vi "Lefoo Atmospheric pressure.vi"(8 "错误输入（无错误）":errorcluster, 11 "VISA resource name":refnum<visa-resource-name> caption="VISA") -> (0 "error out":errorcluster caption="错误输出", 1 "data":string, 2 "Atmospheric pressure":dbl)   [LabVIEW 2017]
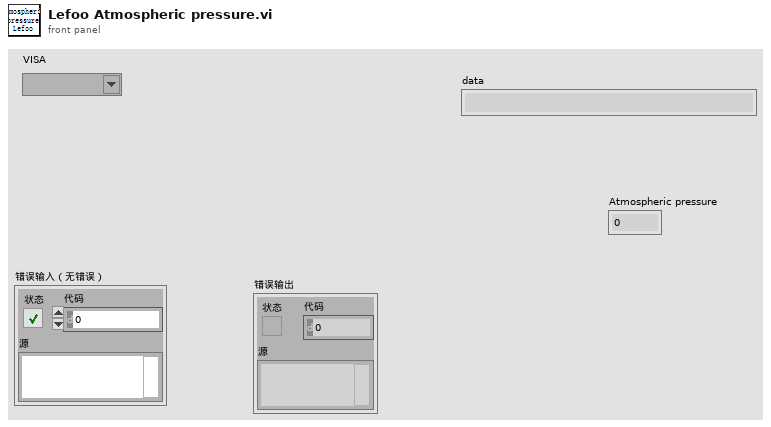
[diagram p1: front panel]
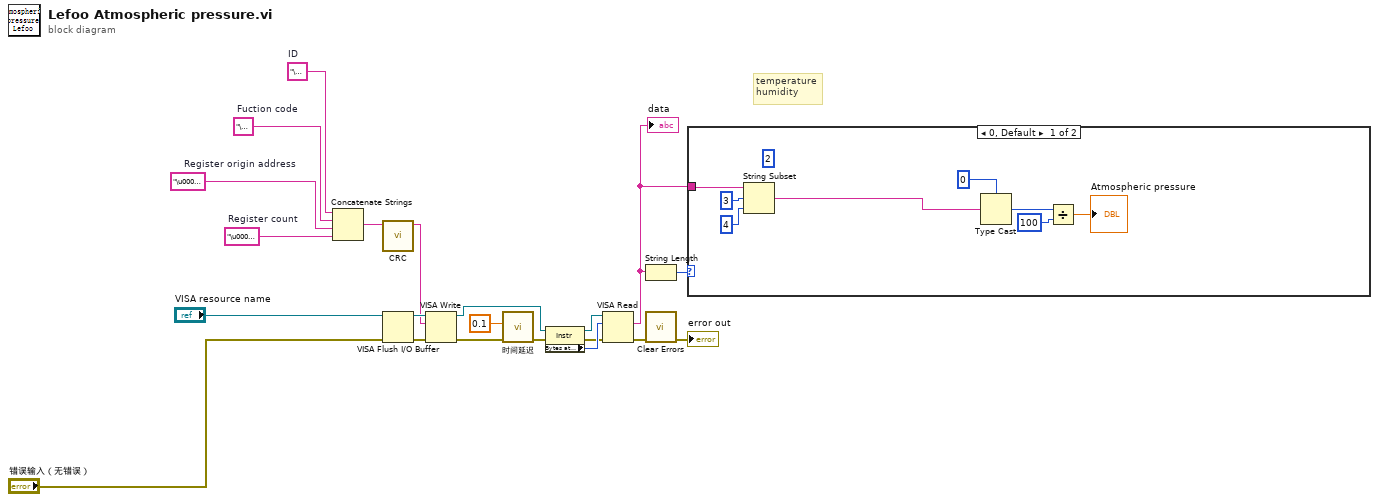
[diagram p0: block diagram]
diagram:
  w2 = "\u0000\u0001"  # Register count
  w4 = "\u0000\u0000"  # Register origin address
  w5 = "\u0003"  # Fuction code
  w6 = "\u0001"  # ID
  # "temperature\nhumidity"
  n1 = Concatenate Strings(w6, w5, w4, w2) -> (w3:string)
  n2 = call "CRC.vi"("字符串"=w3) -> ("连接的字符串"=w14:string)  [unwired: 9 in, 1 out]
  n3 = VISA Flush I/O Buffer(VISA resource name="VISA resource name", error in (no error)="错误输入（无错误）") -> (VISA resource name out=w21:refnum<visa-resource-name>, error out=w19:errorcluster)  [unwired: 1 in]
  n4 = VISA Write(VISA resource name=w21, write buffer=w14, error in (no error)=w19) -> (VISA resource name out=w13:refnum<visa-resource-name>, error out=w20:errorcluster)  [unwired: 1 out]
  n5 = call "时间延迟"("error in (no error)"=w20, "Delay Time (s)"=0.1) -> ("error out"=w11:errorcluster)  [unwired: 9 in]
  n6 = property class="Instr"(reference=w13, error in=w11) -> (reference out=w10:refnum<visa-resource-name>, error out=w9:errorcluster, "Bytes at Port"=w12:u32)
  n7 = VISA Read(VISA resource name=w10, byte count=w12, error in (no error)=w9) -> (read buffer=w8:string, error out=w18:errorcluster)  [unwired: 2 out]
  "data" <- w8
  n8 = String Length(string=w8) -> (length=w7:i32)
  n9 = call <vilib>:"Clear Errors.vi"("error in (no error)"=w18) -> ("error out"=→"error out":errorcluster)  [unwired: 5 in, 1 out]
  n10 = case shown="0, Default" w7 {
    tunnel: w8 -> [w27 _]
    frame 0, Default {
      (unwired) 2
      n11 = String Subset(string=w27, offset (0)=3 ("偏移量(0)"), length (rest)=4 ("长度（剩余）")) -> (substring=w22:string)
      n12 = Type Cast(type=i16 0 ("lo(x) 2"), x=w22) -> (*(type *) &x=w25:i16)
      n13 = Divide(x=w25, y=i16 100) -> (x/y=→"Atmospheric pressure":dbl)
    }
    frame 5 {
    }
  }
